vi "Handle Input.vi"(8 "error in (no error)":errorcluster, 11 "Plugin_Controller in":refnum<class "Plugin_Controller.lvclass">) -> (0 "error out":errorcluster, 3 "Plugin_Controller out":refnum<class "Plugin_Controller.lvclass">)   [LabVIEW 2020, in "Plugin.lvlib" / "Plugin_Controller.lvclass"]
doc: "Reads the measurement data."
uses:
  Plugin_Controller.lvclass
  C:/SVN_LabSys/labsys_lvcode/LabSys_SourceCode/builds/Libraries/LabSys Framework.lvlibp/Configurable Data Node/Configurable Data Node/Configurable Data Node.lvclass
  C:/SVN_LabSys/labsys_lvcode/LabSys_SourceCode/builds/Libraries/LabSys Framework.lvlibp/Data Node/Data Node/Data Node.lvclass
  builds/Libraries/LabSys Framework.lvlibp/Data Distributor/Data Distributor/Value Update.ctl
  builds/Libraries/LabSys Framework.lvlibp/Data Distributor/Value/Value.lvclass
  builds/Libraries/Value Object Library.lvlibp/Double/Double.lvclass
  C:/SVN_LabSys/labsys_lvcode/LabSys_SourceCode/builds/Libraries/LabSys Framework.lvlibp/Data Distributor/Value/Value.lvclass
  builds/Libraries/LabSys Framework.lvlibp/Data Distributor/Value/Value Status.ctl
  Channels/Input Channels/Input Channels.lvclass
  C:/SVN_LabSys/labsys_lvcode/LabSys_SourceCode/Plugin Template/Source/Code/Channels/Plugin_Channels.lvclass
  builds/Libraries/LabSys Framework.lvlibp/Configurable Data Node/Configurable Data Node/Read Module Configuration.vi
  builds/Libraries/LabSys Framework.lvlibp/Data Node/Data Node/Read Error Manager.vi
  builds/Libraries/LabSys Framework.lvlibp/Configuration Storage/Module Configuration/Read Module Name.vi
  builds/Libraries/Value Object Library.lvlibp/Double/Write Value.vi
  builds/Libraries/LabSys Framework.lvlibp/Data Distributor/Value/Write Status.vi
  builds/Libraries/LabSys Framework.lvlibp/Data Distributor/Value/Write Time Stamp.vi
  Plugin_Driver/Plugin_Driver.lvclass
  builds/Libraries/LabSys Framework.lvlibp/Configuration Storage/Module Configuration/Module Configuration.lvclass
  builds/Libraries/LabSys Framework.lvlibp/Error Manager/Error Manager/Error Manager.lvclass
  UI_Class/Plugin_UI.lvclass
  builds/Libraries/LabSys Framework.lvlibp/Data Distributor/Data Distributor/Data Distributor.lvclass
  builds/Libraries/LabSys Framework.lvlibp/Data Node/Data Node/Data Node.lvclass
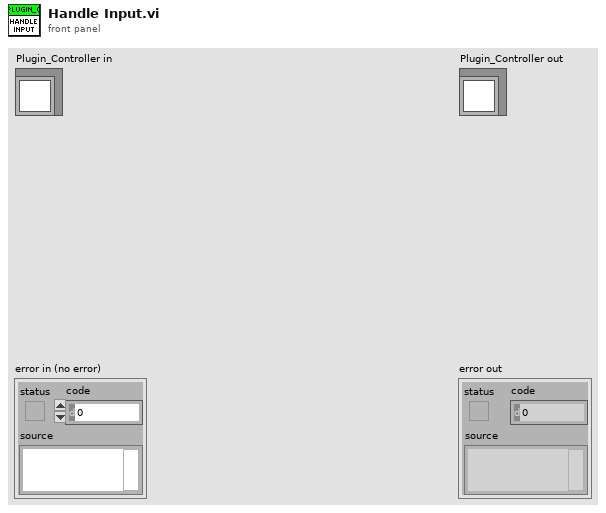
[diagram p1: front panel]
types:
  T1 = typedef "LabSys Framework.lvlibp/Data Distributor.lvlib/Data Distributor.lvclass/Value Update.ctl" = cluster{"Variable Name":string, "Value":refnum<class "Value.lvclass">}
  T2 = typedef "LabSys Framework.lvlibp/Data Distributor.lvlib/Value.lvclass/Value Status.ctl" = enum8{"FAIL", "OK", "UNDEFINED"}
  T3 = typedef "LabSys Framework.lvlibp/Configuration Storage.lvlib/Test Configuration.lvclass/Scaling Information.ctl" = cluster{"Active":bool, "Scaling Type":T4, "Output Minimum":dbl, "Output Maximum":dbl, "Raw Minimum":dbl, "Raw Maximum":dbl, "Output Unit":string, "Function":string, "Lookup Table":string}
  T4 = typedef "LabSys Framework.lvlibp/Configuration Storage.lvlib/Test Configuration.lvclass/Scaling Types.ctl" = enum8{"Linear", "Function", "Lookup Table"}
  T5 = typedef "Plugin Instrument Driver.lvlib/Instrument Driver.lvclass/Measurement Results.ctl" = cluster{"Voltage (V)":dbl}
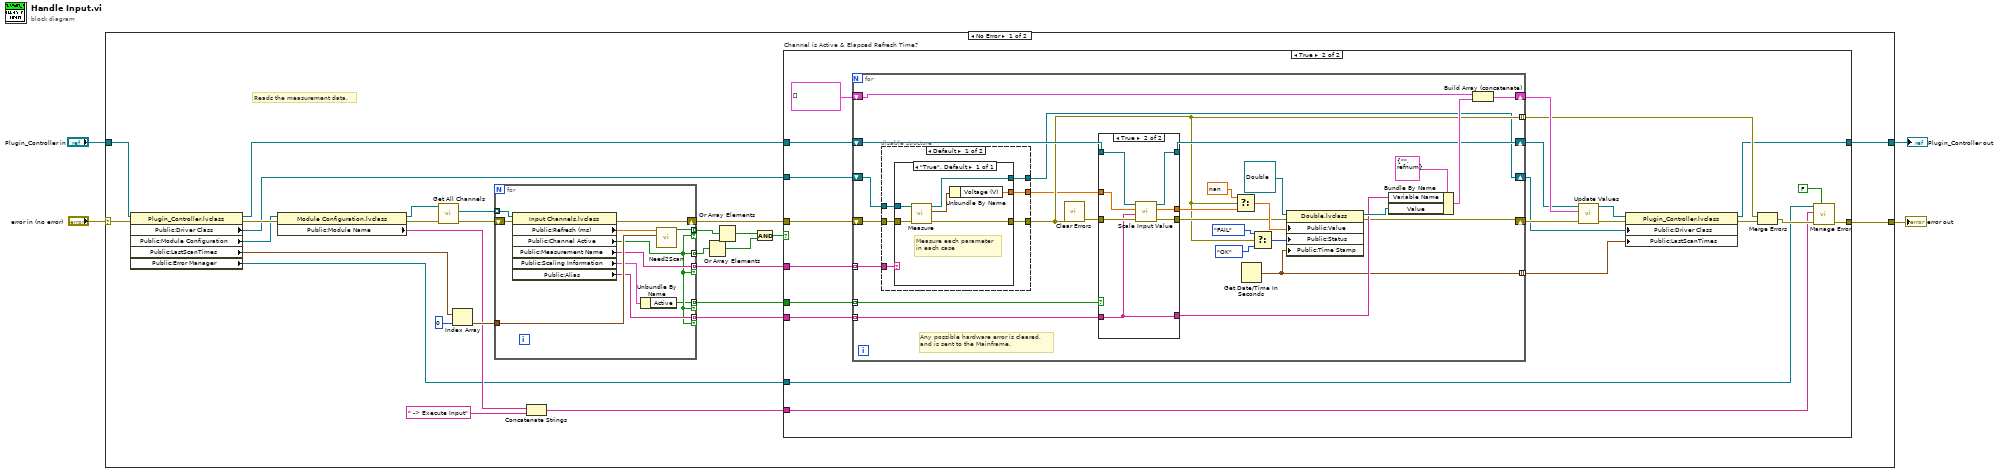
[diagram p0: block diagram]
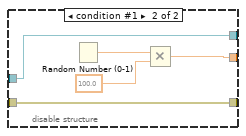
[diagram p3: hidden frame]
diagram:
  n1 = case shown="No Error" "error in (no error)" {
    selector: "error in (no error)" -> [w27 w123]
    tunnel: [w6 w124] -> w2
    tunnel: "Plugin_Controller in" -> [w28 w124]
    tunnel: [w7 w123] -> w1
    frame No Error {
      # "Reads the measurement data."
      n2 = property on="Property Node" class="Plugin_Controller.lvclass"(reference=w28, error in=w27) -> (reference out=w10:refnum<class "Plugin_Controller.lvclass">, error out=w30:errorcluster, "Public:Driver Class"=w13:refnum<class "Plugin_Driver.lvclass">, "Public:Module Configuration"=w29:refnum<class "Module Configuration.lvclass">, "Public:LastScanTimes"=w31:timestamp[], "Public:Error Manager"=w9:refnum<data-value>)
      n3 = property on="Property Node" class="Module Configuration.lvclass"(reference=w29, error in=w30) -> (reference out=w26:refnum<class "Module Configuration.lvclass">, error out=w25:errorcluster, "Public:Module Name"=w16:string)
      n4 = call "Get All Channels.vi"("error in (no error)"=w25, "Module Configuration"=w26) -> ("error out"=w20:errorcluster, "Input Channels[]"=w19:refnum<class "Input Channels.lvclass">[])  [unwired: 5 in, 3 out]
      n5 = Index Array(array=w31, index=0) -> (element=w18:timestamp)
      n6 = for {
        tunnel: w19 -> [w122] mode=indexing
        shift-right: [w120] -> w14
        shift-left: w20 -> [w119]
        tunnel: [w118] -> w24 mode=indexing if=w114
        tunnel: [w114] -> w22 mode=indexing
        tunnel: w18 -> [w117]
        tunnel: [w116] -> w11 mode=indexing if=w114
        tunnel: [w115] -> w12 mode=indexing if=w114
        tunnel: [w113] -> w5 mode=indexing if=w114
        n7 = property on="Property Node" class="Input Channels.lvclass"(reference=w122, error in=w119) -> (error out=w120:errorcluster, "Public:Refresh (ms)"=w121:dbl, "Public:Channel Active"=w114:bool, "Public:Measurement Name"=w115:string, "Public:Scaling Information"=w112:T3, "Public:Alias"=w116:string)  [unwired: 1 out]
        n8 = Unbundle By Name(w112) -> ("Active"=w113:bool)
        n9 = call "Need2Scan.vi"("Time Stamp"=w117, "Refresh (ms)"=w121) -> ("Scan?"=w118:bool)  [unwired: 9 in]
      }
      n10 = Concatenate Strings(w16, " -> Execute Input" ("Error Location")) -> (w8:string)
      n11 = Or Array Elements(Boolean array=w22) -> (logical OR=w21:bool)
      n12 = Or Array Elements(Boolean array=w24) -> (logical OR=w23:bool)
      n13 = And(x=w23, y=w21) -> (x .and. y?=w15:bool)
      n14 = case "Channel is Active & Elapsed Refresh Time?" shown="True" w15 {
        tunnel: w14 -> [w33 w51]
        tunnel: w13 -> [_ w56]
        tunnel: w12 -> [_ w55]
        tunnel: w11 -> [_ w54]
        tunnel: w10 -> [w34 w53]
        tunnel: w9 -> [_ w40]
        tunnel: w8 -> [_ w39]
        tunnel: [w33 w37] -> w7
        tunnel: [w34 w36] -> w6
        tunnel: w5 -> [_ w35]
        frame False {
        }
        frame True {
          n15 = for {
            tunnel: w55 -> [w82] mode=indexing
            tunnel: w54 -> [w80] mode=indexing
            shift-right: [w66] -> w48
            shift-left: w53 -> [w79]
            shift-right: [w65] -> w49
            shift-left: T1[] [] -> [w64]
            tunnel: [w63] -> w42 mode=indexing
            shift-right: [w62] -> w50
            shift-left: w51 -> [w61]
            tunnel: [w60] -> w45 mode=indexing
            shift-right: [w59] -> w44
            shift-left: w56 -> [w83]
            tunnel: w35 -> [w58] mode=indexing
            # "Any possible hardware error is cleared,\nand is sent to the Mainframe."
            n16 = disable-structure shown="Default" {
              disable-tunnel: w83 -> [w89 w96]
              disable-tunnel: w82 -> [w88 _]
              disable-tunnel: [w87 w97] -> w63
              disable-tunnel: w61 -> [w86 w97]
              disable-tunnel: [w85 w96] -> w59
              disable-tunnel: [w84 w98] -> w57
              frame condition #0 (active) {
                n17 = case shown="\"True\", Default" w88 {
                  tunnel: w86 -> [w95]
                  tunnel: w89 -> [w94]
                  tunnel: [w93] -> w87
                  tunnel: [w92] -> w85
                  tunnel: [w90] -> w84
                  frame "True", Default {
                    # "Measure each parameter\nin each case"
                    n18 = call "Measure.vi"("error in"=w95, "Plugin_Driver in"=w94) -> ("error out"=w93:errorcluster, "Measurement Results"=w91:T5, "Plugin_Driver out"=w92:refnum<class "Plugin_Driver.lvclass">)  [unwired: 7 in]
                    n19 = Unbundle By Name(w91) -> ("Voltage (V)"=w90:dbl)
                  }
                }
              }
              frame condition #1 {
                n20 = Random Number (0-1)() -> (number: 0 to 1=w100:dbl)
                n21 = Multiply(x=w100, y=100.0) -> (x*y=w98:dbl)
              }
            }
            n22 = call <vilib>:"Clear Errors.vi"("error in (no error)"=w63) -> ("error out"=w81:errorcluster)  [unwired: 5 in, 1 out]
            n23 = case shown="True" w58 {
              tunnel: w79 -> [w104 w111]
              tunnel: [w104 w110] -> w66
              tunnel: [w101 w109] -> w68
              tunnel: [w103 w108] -> w69
              tunnel: w80 -> [w102 w106]
              tunnel: w81 -> [w103 w107]
              tunnel: [w102 w106] -> w67
              tunnel: w57 -> [w101 w105]
              frame False {
              }
              frame True {
                n24 = call-dynamic "Scale Input Value.vi"("error in (no error)"=w107, "Variable Name"=w106, "Raw Value"=w105, "Configurable Data Node in"=w111) -> ("error out"=w108:errorcluster, "Scaled Value"=w109:dbl, "Configurable Data Node out"=w110:refnum<class "Plugin_Controller.lvclass">)  [unwired: 5 in]
              }
            }
            n25 = Select(t=nan, s=w63, f=w68) -> (s? t:f=w71:dbl)
            n26 = Get Date/Time In Seconds() -> (seconds since 1Jan1904=w60:timestamp)
            n27 = Select(t=Value_Status."FAIL" ("Status"), s=w63, f=Value_Status."OK" ("Status")) -> (s? t:f=w72:T2)
            n28 = property on="Property Node" class="Double.lvclass"(reference=refnum<class "Double.lvclass"> refnum ("Value Object Library.lvlibp:Double.lvclass"), error in=w69, "Public:Value"=w71, "Public:Status"=w72, "Public:Time Stamp"=w60) -> (reference out=w77:refnum<class "Double.lvclass">, error out=w62:errorcluster)
            n29 = Bundle By Name(cluster=T1 {"Variable Name"="", "Value"=refnum} ("Value Update"), "Variable Name"=w67, "Value"=w77) -> (w76:T1)
            n30 = Build Array (concatenate)(w64, w76) -> (w65:T1[])
          }
          n31 = call "Update Values.vi"("error in (no error)"=w50, "Value Updates"=w49, "Data Node in"=w48) -> ("error out"=w46:errorcluster, "Data Node out"=w47:refnum<class "Plugin_Controller.lvclass">)  [unwired: 7 in]
          n32 = property class="Plugin_Controller.lvclass"(reference=w47, error in=w46, "Public:Driver Class"=w44, "Public:LastScanTimes"=w45) -> (reference out=w36:refnum<class "Plugin_Controller.lvclass">, error out=w43:errorcluster)
          n33 = Merge Errors(w42, w43) -> (w41:errorcluster)
          n34 = call "Manage Error.vi"("Clear Errors (F)"=FALSE, "error in (no error)"=w41, "Error Location"=w39, "Error Manager in"=w40) -> ("error out"=w37:errorcluster)  [unwired: 6 in, 1 out]
        }
      }
    }
    frame Error {
    }
  }
  "error out" <- w1
  "Plugin_Controller out" <- w2
